vi "Set Power Setpoints.vi"(8 "error in (no error)":errorcluster, 9 "Right Power Setpoint":dbl(slide) min=-1.0 max=1.0 step=0.1 scale=-1.0..1.0, 10 "Left Power Setpoint":dbl(slide) min=-1.0 max=1.0 step=0.1 scale=-1.0..1.0, 11 "Drive Train in":refnum<class "Drive Train.lvclass">) -> (0 "error out":errorcluster, 3 "Drive Train out":refnum<class "Drive Train.lvclass">)   [LabVIEW 2014, in "Logical Systems.lvlib" / "Drive Train.lvlib" / "Drive Train.lvclass"]
uses:
  Drive Train.lvclass
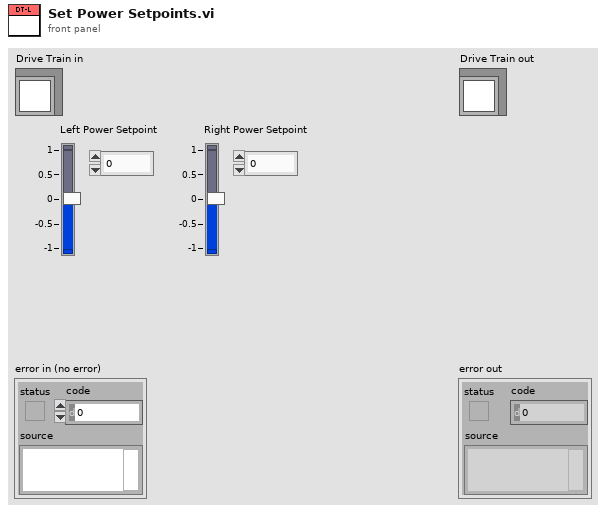
[diagram p1: front panel]
types:
  T1 = typedef "Logical Systems.lvlib/Drive Train.lvlib/Drive Train.lvclass/Drive Train Status.ctl" = cluster{"Left Power":dbl, "Right Power":dbl, "Left Power Setpoint":dbl, "Right Power Setpoint":dbl}
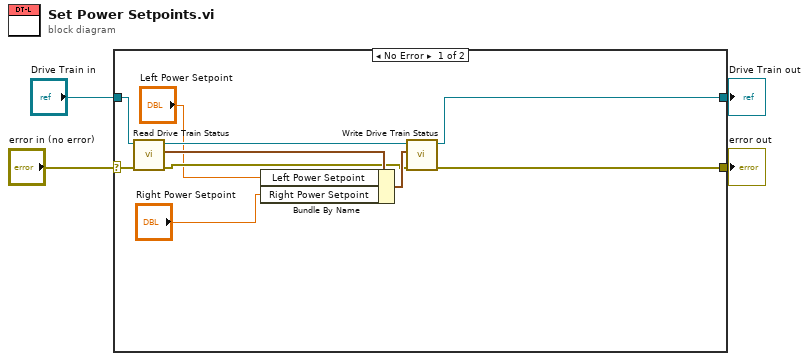
[diagram p0: block diagram]
diagram:
  n1 = case shown="No Error" "error in (no error)" {
    selector: "error in (no error)" -> [w8 w16]
    tunnel: [w6 w16] -> w3
    tunnel: [w12 w15] -> w1
    tunnel: "Drive Train in" -> [w13 w15]
    frame No Error {
      n2 = call-dynamic "Read Drive Train Status.vi"("error in (no error)"=w8, "Drive Train in"=w13) -> ("error out"=w7:errorcluster, "Drive Train Status"=w11:T1, "Drive Train out"=w14:refnum<class "Drive Train.lvclass">)  [unwired: 7 in]
      n3 = Bundle By Name(cluster=w11, "Left Power Setpoint"="Left Power Setpoint", "Right Power Setpoint"="Right Power Setpoint") -> (w10:T1)
      n4 = call-dynamic "Write Drive Train Status.vi"("error in (no error)"=w7, "Drive Train Status"=w10, "Drive Train in"=w14) -> ("error out"=w6:errorcluster, "Drive Train out"=w12:refnum<class "Drive Train.lvclass">)  [unwired: 7 in]
    }
    frame Error {
    }
  }
  "error out" <- w3
  "Drive Train out" <- w1
